vi "Close.vi"(8 "error in (no error)":errorcluster, 11 "NI Digitizer in":refnum<class "NI Digitizer.lvclass">) -> (0 "error out":errorcluster, 3 "NI Digitizer out":refnum<class "NI Digitizer.lvclass">)   [LabVIEW 2025, in "Digitizer.lvlib" / "NI Digitizer.lvclass"]
uses:
  NI Digitizer.lvclass
  NI Digitizer.lvclass/NI Digitizer.ctl
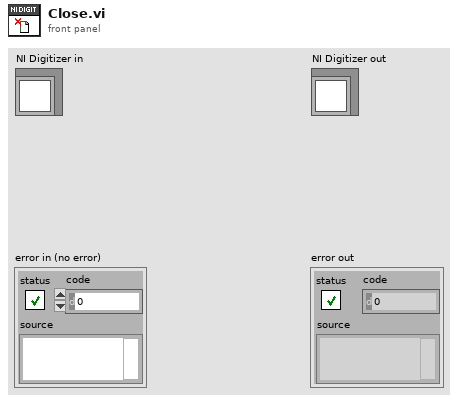
[diagram p1: front panel]
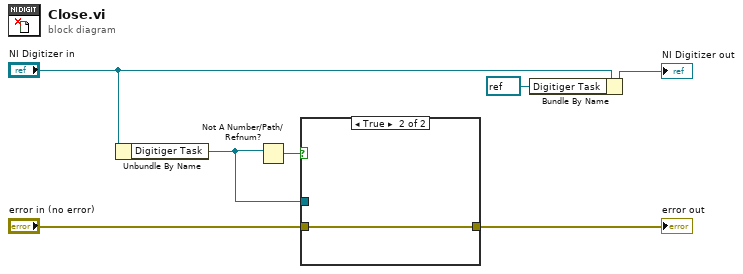
[diagram p0: block diagram]
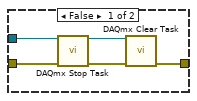
[diagram p2: hidden frame]
diagram:
  n1 = Unbundle By Name("NI Digitizer in") -> ("Digitiger Task"=w5:refnum<k21>)
  n2 = Not A Number/Path/Refnum?(number/path/refnum=w5) -> (NaN/Path/Refnum?=w6:bool)
  n3 = case shown="True" w6 {
    tunnel: [w12 w13] -> w1
    tunnel: "error in (no error)" -> [w11 w13]
    tunnel: w5 -> [w8 _]
    frame False {
      n4 = call <vilib>:"DAQmx Stop Task.vi"("task/channels in"=w8, "error in"=w11) -> ("task out"=w9:refnum<k21>, "error out"=w10:errorcluster)  [unwired: 12 in]
      n5 = call <vilib>:"DAQmx Clear Task.vi"("task in"=w9, "error in"=w10) -> ("error out"=w12:errorcluster)  [unwired: 13 in]
    }
    frame True {
    }
  }
  "error out" <- w1
  n6 = Bundle By Name(cluster="NI Digitizer in", "Digitiger Task"=refnum<k21> refnum) -> (→"NI Digitizer out":refnum<class "NI Digitizer.lvclass">)
